vi "Boolean To TF.vi"(4 "Boolean":bool) -> (1 "mso bool":i32)   [LabVIEW 2020, in "lvpptx.lvlib"]
uses:
  lvpptx.lvlib
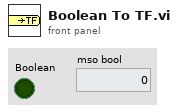
[diagram p1: front panel]
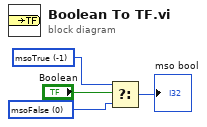
[diagram p0: block diagram]
diagram:
  w2 = -1 items=["msoTrue"=-1, "msoFalse"=0, "msoCTrue"=1, "msoTriStateToggle"=-3, "msoTriStateMixed"=-2] ("Bold")
  w3 = 0 items=["msoTrue"=-1, "msoFalse"=0, "msoCTrue"=1, "msoTriStateToggle"=-3, "msoTriStateMixed"=-2] ("Bold")
  n1 = Select(t=w2, s="Boolean", f=w3) -> (s? t:f=→"mso bool":i32)
